vi "chart series set error bars direction.vi"(8 "error in (no error)":errorcluster, 10 "direction":u8, 11 "error_bars":u32) -> (0 "error out":errorcluster)   [LabVIEW 8.6]
doc: "void chart_series_set_error_bars_direction(lxw_series_error_bars error_bars, uint8_t direction);"
uses:
  pending_lvxlsxwriter/xlsxwriter.dll
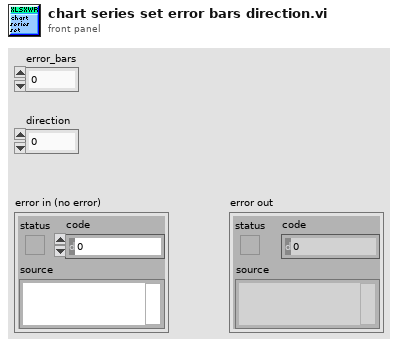
[diagram p1: front panel]
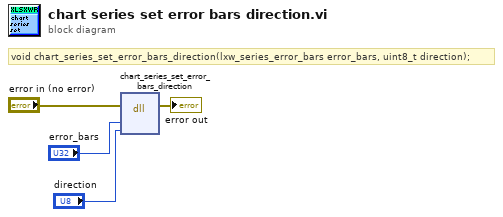
[diagram p0: block diagram]
diagram:
  # "void chart_series_set_error_bars_direction(lxw_series_error_bars error_bars, uint8_t direction);"
  n1 = dll-call lib="C:/Users/WDAGUtilityAccount/Desktop/pending_lvxlsxwriter/xlsxwriter.*" fn="chart_series_set_error_bars_direction"(error in="error in (no error)", "error_bars"="error_bars", "direction"="direction") -> (error out=→"error out":errorcluster)  [unwired: 5 in, 1 out]
